vi "Dispose.vi"(8 "error in (no error)":errorcluster, 11 "Disposable in":refnum<data-value>) -> (0 "error out":errorcluster)   [LabVIEW 2020, in "Lua for LabVIEW.lvlib" / "Disposable.lvclass"]
uses:
  Disposable.lvclass
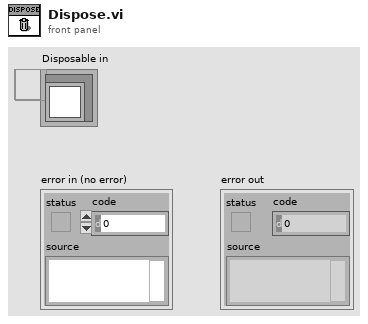
[diagram p1: front panel]
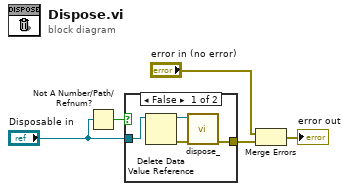
[diagram p0: block diagram]
diagram:
  n1 = Not A Number/Path/Refnum?(number/path/refnum="Disposable in") -> (NaN/Path/Refnum?=w5:bool)
  n2 = case shown="False" w5 {
    tunnel: "Disposable in" -> [w9 _]
    tunnel: [w6 _] -> w2
    frame False {
      n3 = Delete Data Value Reference(data value reference=w9) -> (data value=w8:refnum<class "Disposable.lvclass">, error out=w7:errorcluster)  [unwired: 1 in]
      n4 = call-dynamic "dispose_.vi"("error in (no error)"=w7, "Disposable in"=w8) -> ("error out"=w6:errorcluster)  [unwired: 9 in]
    }
    frame True {
    }
  }
  n5 = Merge Errors("error in (no error)", w2) -> (→"error out":errorcluster)
